vi "Get BLISS_Fingerprint Log.vi"(7 "Action":enum16{"Server Access", "File Access"}(ring), 8 "error in (no error)":errorcluster, 9 "size (in bytes)":i64, 10 "source filepath":path, 11 "Data Parameters in":T1) -> (0 "error out":errorcluster)   [LabVIEW 2020]
uses:
  MC5e Gobal_Variables.vi
  MC5e Squad_Info.ctl
  MC5e Unit_Status_List.ctl
  MC5e Data_Parameters.ctl
  MC5e Terrain types.ctl
  Location.ctl
  MC5e Unit.ctl
  MC5e Force.ctl
panel:
  in  "error in":errorcluster
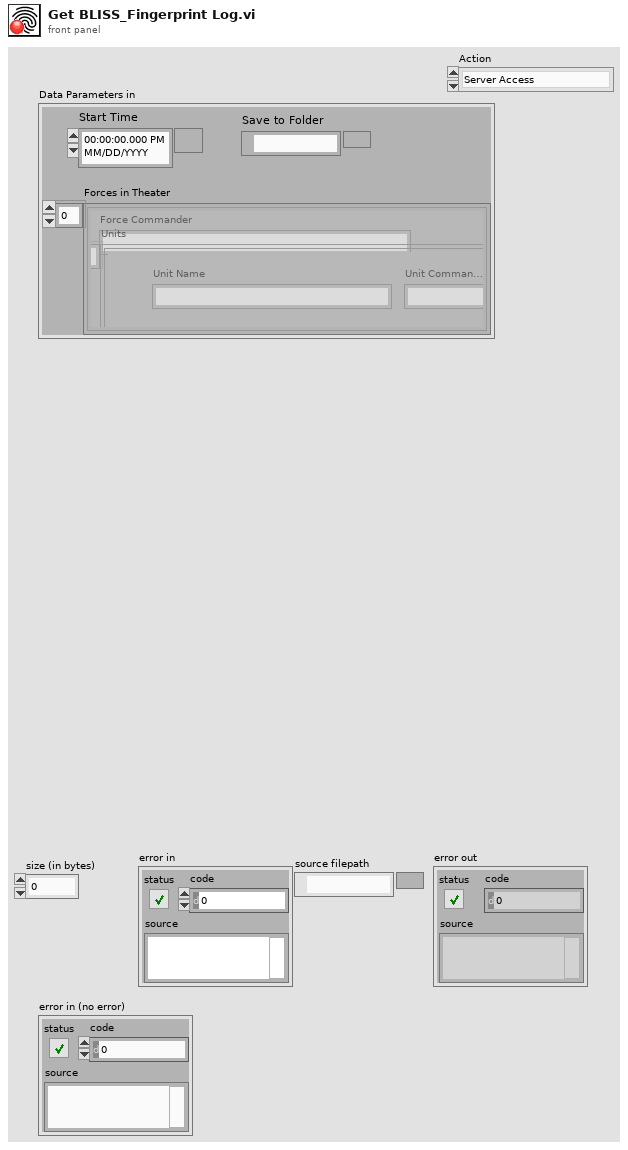
[diagram p1: front panel]
types:
  T1 = typedef "MC5e Data_Parameters.ctl" = cluster{"Start Time":timestamp, "Save to Folder":path, "Forces in Theater":T2[]}
  T2 = typedef "MC5e Force.ctl" = cluster{"Force Commander":string, "Units":T3[]}
  T3 = typedef "MC5e Unit.ctl" = cluster{"Squad List":T4, "Unit Fatigue Level":enum16{"Not Fatigued", "Fatigued", "Seriously Fatigued"}, "Flying Unit":bool, "Mounted Unit":bool, "Difficult Terrain Types":T6, "Full BR":dbl, "Defending from Stronghold":bool, "Speed":dbl, "Capacity %":dbl, "Morale":dbl, "Current BR":dbl, "Location":T7, "Unit Name":string, "Unit Commander":string, "Unit Notes":string}
  T4 = typedef "MC5e Unit_Status_List.ctl" = T5[]
  T5 = typedef "MC5e Squad_Info.ctl" = cluster{"Squad Name":string, "# Soldiers":dbl, "Battle Rating":dbl, "Flying":bool, "Mounted":bool, "Speed":dbl, "Range":dbl, "Morale":dbl, "Token Image":variant, "Max Endurance":dbl, "Current Endurance":dbl, "Difficult Terrain":T6}
  T6 = typedef "MC5e Terrain types.ctl" = cluster{"Artic / snow / ice)":bool, "Coast":bool, "Desert / sand":bool, "Forest / woodland":bool, "Grassland / plains":bool, "Mountain / canyons":bool, "Underdark / caverns":bool, "Acquatic / rivers, lakes, ocean":bool}
  T7 = typedef "Location.ctl" = cluster{"X coordinate":dbl, "Y coordinate":dbl}
  T8 = enum16{"open", "replace", "create", "open or create", "replace or create", "replace or create with confirmation"}
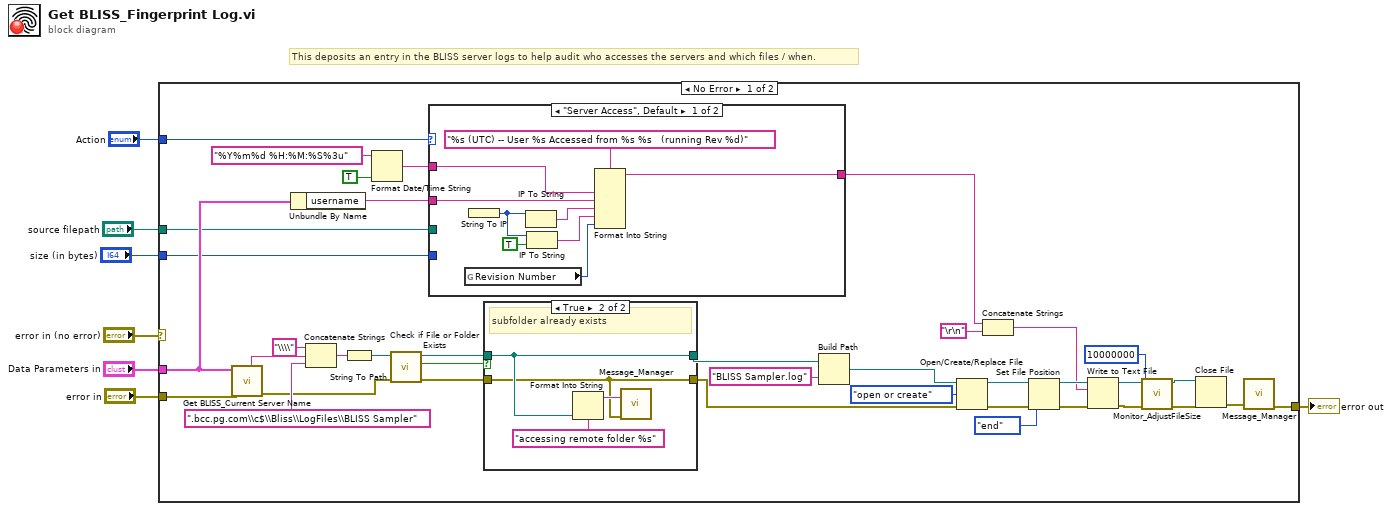
[diagram p0: block diagram]
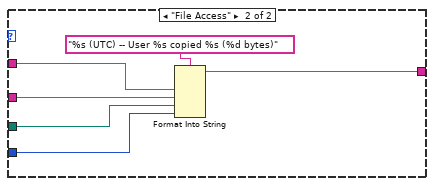
[diagram p2: hidden frame]
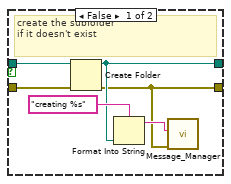
[diagram p3: hidden frame]
diagram:
  # "This deposits an entry in the BLISS server logs to help audit who accesses the servers and which files / when."
  n1 = case shown="No Error" "error in (no error)" {
    tunnel: "Action" -> [w22 _]
    tunnel: "Data Parameters in" -> [w19 _]
    tunnel: "error in" -> [w23 w71]
    tunnel: [w10 w71] -> w3
    tunnel: "source filepath" -> [w9 _]
    tunnel: "size (in bytes)" -> [w8 _]
    frame No Error {
      n2 = call "Get BLISS_Current Server Name.vi"("error in"=w23, "Data Parameters in"=w19) -> ("error out"=w24:errorcluster, "Server Name"=w25:string)  [unwired: 6 in, 2 out]
      n3 = Unbundle By Name(w19) -> ("username"=w18:string)
      n4 = Concatenate Strings("\\\\" ("string"), w25, ".bcc.pg.com\\c$\\Bliss\\LogFiles\\BLISS Sampler" ("string")) -> (w28:string)
      n5 = String To Path(string=w28) -> (path=w27:path)
      n6 = Format Date/Time String(time format string (%c)="%Y%m%d %H:%M:%S%3u", UTC format=TRUE) -> (date/time string=w17:string)  [unwired: 1 in]
      n7 = call <vilib>:"Check if File or Folder Exists.vi"("error in (no error)"=w24, "path"=w27) -> ("error out"=w29:errorcluster, "file or folder exists?"=w31:bool, "dup path"=w30:path)  [unwired: 7 in]
      n8 = case shown="\"Server Access\", Default" w22 {
        tunnel: w18 -> [w47 w57]
        tunnel: w17 -> [w48 w58]
        tunnel: [w49 w59] -> w16
        tunnel: w9 -> [_ w56]
        tunnel: w8 -> [_ w55]
        frame "Server Access", Default {
          n9 = global read "MC5e Gobal_Variables.vi" "Revision Number"() -> (w46:i32)
          n10 = String To IP() -> (0:w53:u32)  [unwired: 1 in]
          n11 = IP To String(2:w53) -> (0:w51:string)  [unwired: 1 in]
          n12 = IP To String(1:TRUE ("dot notation? (F)"), 2:w53) -> (0:w50:string)
          n13 = Format Into String(format string="%s (UTC) -- User %s Accessed from %s %s   (running Rev %d)", w48, w47, w51, w50, w46) -> (resulting string=w49:string)  [unwired: 2 in, 1 out]
        }
        frame "File Access" {
          n14 = Format Into String(format string="%s (UTC) -- User %s copied %s (%d bytes)", w58, w57, w56, w55) -> (resulting string=w59:string)  [unwired: 2 in, 1 out]
        }
      }
      n15 = case shown="True" w31 {
        tunnel: w30 -> [w66 w69]
        tunnel: w29 -> [w65 w67]
        tunnel: [w61 w67] -> w12
        tunnel: [w62 w69] -> w15
        frame False {
          # "create the subfolder\nif it doesn't exist"
          n16 = Create Folder(path (use dialog)=w66, error in=w65) -> (created path=w62:path, error out=w61:errorcluster)  [unwired: 1 in, 1 out]
          n17 = Format Into String(format string="creating %s", w62) -> (resulting string=w64:string)  [unwired: 2 in, 1 out]
          n18 = call "Message_Manager.vi"("error in"=w61, "New Entry"=w64) -> ()  [unwired: 4 in, 6 out]
        }
        frame True {
          # "subfolder already exists"
          n19 = Format Into String(format string="accessing remote folder %s", w69) -> (resulting string=w68:string)  [unwired: 2 in, 1 out]
          n20 = call "Message_Manager.vi"("error in"=w67, "New Entry"=w68) -> ()  [unwired: 4 in, 6 out]
        }
      }
      n21 = Build Path(base path=w15, name or relative path="BLISS Sampler.log" ("string")) -> (appended path=w13:path)
      n22 = Open/Create/Replace File(file path (use dialog)=w13, error in=w12, operation (0:open)=T8."open or create") -> (refnum out=w40:refnum<file>, error out=w39:errorcluster)  [unwired: 3 in, 1 out]
      n23 = Concatenate Strings(w16, "\r\n") -> (w33:string)
      n24 = Set File Position(refnum=w40, from (0:start)=enum16{"start", "end", "current"}."end", error in=w39) -> (refnum out=w42:refnum<file>, error out=w41:errorcluster)  [unwired: 1 in]
      n25 = Write to Text File(file (use dialog)=w42, text=w33, error in=w41) -> (refnum out=w38:refnum<file>, error out=w37:errorcluster)  [unwired: 1 in, 1 out]
      n26 = call "Monitor_AdjustFileSize.vi"("Error In"=w37, "Max File Size in Bytes"=i64 10000000, "Refnum In"=w38) -> ("Error Out"=w36:errorcluster, "Refnum Out"=w35:refnum<file>)  [unwired: 5 in, 2 out]
      n27 = Close File(refnum=w35, error in=w36) -> (error out=w11:errorcluster)  [unwired: 1 out]
      n28 = call "Message_Manager.vi"("error in"=w11) -> ("error out"=w10:errorcluster)  [unwired: 5 in, 5 out]
    }
    frame Error {
    }
  }
  "error out" <- w3
